vi "Main.vi"() -> ()   [LabVIEW 2013]
uses:
  ctl/config_ctl.ctl
  ctl/force_sensor_data.ctl
  ctl/UI_cmd-ctl.ctl
  ctl/file_path-cmd.ctl
  ctl/Data_analysis_mune_index.ctl
  <vilib>/Analysis/baseanly.llb/Mean (DBL).vi
  Global.vi
  <vilib>/Utility/file.llb/Read From Spreadsheet File (string).vi
  <vilib>/Analysis/NI_AALBase.lvlib
panel:
  out "simulation":bool=TRUE
  in  "sub_tab":enum32{"graph", "ref", "err"}(tab)=enum."ref"
  in  "Grapb_tap":enum32{"data graph", "sub graph"}(tab)=enum."sub graph"
  out "Strain chart w cal":waveform(dbl)[](graph)
  out "Force chart":waveform(dbl)(graph)
  out "vacuum chart":waveform(dbl)(graph)
  out "Heater chart":i32(graph)=2147483647
  out "Strain raw chart":waveform(dbl)[](graph)=[{"t0"=timestamp(3479370102.41062 s since 1904-01-01), "dt"=0.00062, "Y"=[0.0, 0.0, 0.0, 0.0, 0.0, 0.0, 0.0, 0.0, 0.0, 0.0, 0.0, 0.0, 0.0, 0.0, 0.0, 0.0, 0.0, 0.0, 0.0, 0.0, 0.0, 0.0, 0.0, 0.0, 0.0, 0.0, 0.0, 0.0, 0.0, 0.0, 0.0, 0.0, 0.0, 0.0, 0.0, 0.0, 0.0, 0.0, 0.0, 0.0, 0.0, 0.0, 0.0, 0.0, 0.0, 0.0, 0.0, 0.0, 0.0, 0.0, 0.0, 0.0, 0.0, 0.0, 0.0, 0.0, 0.0, 0.0, 0.0, 0.0, 0.0, 0.0, 0.0, 0.0, 0.0, 0.0, 0.0, 0.0, 0.0, 0.0, 0.0, 0.0, 0.0, 0.0, 0.0, 0.0, 0.0, 0.0, 0.0, 0.0, 0.0, 0.0, 0.0, 0.0, 0.0, 0.0, 0.0, 0.0, 0.0, 0.0, 0.0, 0.0, 0.0, 0.0, 0.0, 0.0, 0.0, 0.0, 0.0, 0.0], "attributes"=variant("NI_ChannelName"=variant(string "변형률_0"), "NI_UnitDescription"=variant(string "Strain"))}, {"t0"=timestamp(3479370102.41062 s since 1904-01-01), "dt"=0.00062, "Y"=[0.0, 0.0, 0.0, 0.0, 0.0, 0.0, 0.0, 0.0, 0.0, 0.0, 0.0, 0.0, 0.0, 0.0, 0.0, 0.0, 0.0, 0.0, 0.0, 0.0, 0.0, 0.0, 0.0, 0.0, 0.0, 0.0, 0.0, 0.0, 0.0, 0.0, 0.0, 0.0, 0.0, 0.0, 0.0, 0.0, 0.0, 0.0, 0.0, 0.0, 0.0, 0.0, 0.0, 0.0, 0.0, 0.0, 0.0, 0.0, 0.0, 0.0, 0.0, 0.0, 0.0, 0.0, 0.0, 0.0, 0.0, 0.0, 0.0, 0.0, 0.0, 0.0, 0.0, 0.0, 0.0, 0.0, 0.0, 0.0, 0.0, 0.0, 0.0, 0.0, 0.0, 0.0, 0.0, 0.0, 0.0, 0.0, 0.0, 0.0, 0.0, 0.0, 0.0, 0.0, 0.0, 0.0, 0.0, 0.0, 0.0, 0.0, 0.0, 0.0, 0.0, 0.0, 0.0, 0.0, 0.0, 0.0, 0.0, 0.0], "attributes"=variant("NI_ChannelName"=variant(string "변형률_1"), "NI_UnitDescription"=variant(string "Strain"))}, {"t0"=timestamp(3479370102.41062 s since 1904-01-01), "dt"=0.00062, "Y"=[0.0, 0.0, 0.0, 0.0, 0.0, 0.0, 0.0, 0.0, 0.0, 0.0, 0.0, 0.0, 0.0, 0.0, 0.0, 0.0, 0.0, 0.0, 0.0, 0.0, 0.0, 0.0, 0.0, 0.0, 0.0, 0.0, 0.0, 0.0, 0.0, 0.0, 0.0, 0.0, 0.0, 0.0, 0.0, 0.0, 0.0, 0.0, 0.0, 0.0, 0.0, 0.0, 0.0, 0.0, 0.0, 0.0, 0.0, 0.0, 0.0, 0.0, 0.0, 0.0, 0.0, 0.0, 0.0, 0.0, 0.0, 0.0, 0.0, 0.0, 0.0, 0.0, 0.0, 0.0, 0.0, 0.0, 0.0, 0.0, 0.0, 0.0, 0.0, 0.0, 0.0, 0.0, 0.0, 0.0, 0.0, 0.0, 0.0, 0.0, 0.0, 0.0, 0.0, 0.0, 0.0, 0.0, 0.0, 0.0, 0.0, 0.0, 0.0, 0.0, 0.0, 0.0, 0.0, 0.0, 0.0, 0.0, 0.0, 0.0], "attributes"=variant("NI_ChannelName"=variant(string "변형률_2"), "NI_UnitDescription"=variant(string "Strain"))}, {"t0"=timestamp(3479370102.41062 s since 1904-01-01), "dt"=0.00062, "Y"=[0.0, 0.0, 0.0, 0.0, 0.0, 0.0, 0.0, 0.0, 0.0, 0.0, 0.0, 0.0, 0.0, 0.0, 0.0, 0.0, 0.0, 0.0, 0.0, 0.0, 0.0, 0.0, 0.0, 0.0, 0.0, 0.0, 0.0, 0.0, 0.0, 0.0, 0.0, 0.0, 0.0, 0.0, 0.0, 0.0, 0.0, 0.0, 0.0, 0.0, 0.0, 0.0, 0.0, 0.0, 0.0, 0.0, 0.0, 0.0, 0.0, 0.0, 0.0, 0.0, 0.0, 0.0, 0.0, 0.0, 0.0, 0.0, 0.0, 0.0, 0.0, 0.0, 0.0, 0.0, 0.0, 0.0, 0.0, 0.0, 0.0, 0.0, 0.0, 0.0, 0.0, 0.0, 0.0, 0.0, 0.0, 0.0, 0.0, 0.0, 0.0, 0.0, 0.0, 0.0, 0.0, 0.0, 0.0, 0.0, 0.0, 0.0, 0.0, 0.0, 0.0, 0.0, 0.0, 0.0, 0.0, 0.0, 0.0, 0.0], "attributes"=variant("NI_ChannelName"=variant(string "변형률_3"), "NI_UnitDescription"=variant(string "Strain"))}]
  out "Strain raw graph":waveform(dbl)[](graph)=[{"t0"=timestamp(3479370102.41062 s since 1904-01-01), "dt"=0.00062, "Y"=[0.04635468247337127, 0.04635468247337127, 0.04635468247337127, 0.04635468247337127, 0.04635468247337127, 0.04635468247337127, 0.04635468247337127, 0.04635468247337127, 0.04635468247337127, 0.04635468247337127, 0.04635468247337127, 0.04635468247337127, 0.04635468247337127, 0.04635468247337127, 0.04635468247337127, 0.04635468247337127, 0.04635468247337127, 0.04635468247337127, 0.04635468247337127, 0.04635468247337127, 0.04635468247337127, 0.04635468247337127, 0.04635468247337127, 0.04635468247337127, 0.04635468247337127, 0.04635468247337127, 0.04635468247337127, 0.04635468247337127, 0.04635468247337127, 0.04635468247337127, 0.04635468247337127, 0.04635468247337127, 0.04635468247337127, 0.04635468247337127, 0.04635468247337127, 0.04635468247337127, 0.04635468247337127, 0.04635468247337127, 0.04635468247337127, 0.04635468247337127, 0.04635468247337127, 0.04635468247337127, 0.04635468247337127, 0.04635468247337127, 0.04635468247337127, 0.04635468247337127, 0.04635468247337127, 0.04635468247337127, 0.04635468247337127, 0.04635468247337127, 0.04635468247337127, 0.04635468247337127, 0.04635468247337127, 0.04635468247337127, 0.04635468247337127, 0.04635468247337127, 0.04635468247337127, 0.04635468247337127, 0.04635468247337127, 0.04635468247337127, 0.04635468247337127, 0.04635468247337127, 0.04635468247337127, 0.04635468247337127, 0.04635468247337127, 0.04635468247337127, 0.04635468247337127, 0.04635468247337127, 0.04635468247337127, 0.04635468247337127, 0.04635468247337127, 0.04635468247337127, 0.04635468247337127, 0.04635468247337127, 0.04635468247337127, 0.04635468247337127, 0.04635468247337127, 0.04635468247337127, 0.04635468247337127, 0.04635468247337127, 0.04635468247337127, 0.04635468247337127, 0.04635468247337127, 0.04635468247337127, 0.04635468247337127, 0.04635468247337127, 0.04635468247337127, 0.04635468247337127, 0.04635468247337127, 0.04635468247337127, 0.04635468247337127, 0.04635468247337127, 0.04635468247337127, 0.04635468247337127, 0.04635468247337127, 0.04635468247337127, 0.04635468247337127, 0.04635468247337127, 0.04635468247337127, 0.04635468247337127], "attributes"=variant("NI_ChannelName"=variant(string "변형률_0"), "NI_UnitDescription"=variant(string "Strain"))}, {"t0"=timestamp(3479370102.41062 s since 1904-01-01), "dt"=0.00062, "Y"=[0.04702815089622699, 0.04702815089622699, 0.04702815089622699, 0.04702815089622699, 0.04702815089622699, 0.04702815089622699, 0.04702815089622699, 0.04702815089622699, 0.04702815089622699, 0.04702815089622699, 0.04702815089622699, 0.04702815089622699, 0.04702815089622699, 0.04702815089622699, 0.04702815089622699, 0.04702815089622699, 0.04702815089622699, 0.04702815089622699, 0.04702815089622699, 0.04702815089622699, 0.04702815089622699, 0.04702815089622699, 0.04702815089622699, 0.04702815089622699, 0.04702815089622699, 0.04702815089622699, 0.04702815089622699, 0.04702815089622699, 0.04702815089622699, 0.04702815089622699, 0.04702815089622699, 0.04702815089622699, 0.04702815089622699, 0.04702815089622699, 0.04702815089622699, 0.04702815089622699, 0.04702815089622699, 0.04702815089622699, 0.04702815089622699, 0.04702815089622699, 0.04702815089622699, 0.04702815089622699, 0.04702815089622699, 0.04702815089622699, 0.04702815089622699, 0.04702815089622699, 0.04702815089622699, 0.04702815089622699, 0.04702815089622699, 0.04702815089622699, 0.04702815089622699, 0.04702815089622699, 0.04702815089622699, 0.04702815089622699, 0.04702815089622699, 0.04702815089622699, 0.04702815089622699, 0.04702815089622699, 0.04702815089622699, 0.04702815089622699, 0.04702815089622699, 0.04702815089622699, 0.04702815089622699, 0.04702815089622699, 0.04702815089622699, 0.04702815089622699, 0.04702815089622699, 0.04702815089622699, 0.04702815089622699, 0.04702815089622699, 0.04702815089622699, 0.04702815089622699, 0.04702815089622699, 0.04702815089622699, 0.04702815089622699, 0.04702815089622699, 0.04702815089622699, 0.04702815089622699, 0.04702815089622699, 0.04702815089622699, 0.04702815089622699, 0.04702815089622699, 0.04702815089622699, 0.04702815089622699, 0.04702815089622699, 0.04702815089622699, 0.04702815089622699, 0.04702815089622699, 0.04702815089622699, 0.04702815089622699, 0.04702815089622699, 0.04702815089622699, 0.04702815089622699, 0.04702815089622699, 0.04702815089622699, 0.04702815089622699, 0.04702815089622699, 0.04702815089622699, 0.04702815089622699, 0.04702815089622699], "attributes"=variant("NI_ChannelName"=variant(string "변형률_1"), "NI_UnitDescription"=variant(string "Strain"))}, {"t0"=timestamp(3479370102.41062 s since 1904-01-01), "dt"=0.00062, "Y"=[0.046751224408544026, 0.046751224408544026, 0.046751224408544026, 0.046751224408544026, 0.046751224408544026, 0.046751224408544026, 0.046751224408544026, 0.046751224408544026, 0.046751224408544026, 0.046751224408544026, 0.046751224408544026, 0.046751224408544026, 0.046751224408544026, 0.046751224408544026, 0.046751224408544026, 0.046751224408544026, 0.046751224408544026, 0.046751224408544026, 0.046751224408544026, 0.046751224408544026, 0.046751224408544026, 0.046751224408544026, 0.046751224408544026, 0.046751224408544026, 0.046751224408544026, 0.046751224408544026, 0.046751224408544026, 0.046751224408544026, 0.046751224408544026, 0.046751224408544026, 0.046751224408544026, 0.046751224408544026, 0.046751224408544026, 0.046751224408544026, 0.046751224408544026, 0.046751224408544026, 0.046751224408544026, 0.046751224408544026, 0.046751224408544026, 0.046751224408544026, 0.046751224408544026, 0.046751224408544026, 0.046751224408544026, 0.046751224408544026, 0.046751224408544026, 0.046751224408544026, 0.046751224408544026, 0.046751224408544026, 0.046751224408544026, 0.046751224408544026, 0.046751224408544026, 0.046751224408544026, 0.046751224408544026, 0.046751224408544026, 0.046751224408544026, 0.046751224408544026, 0.046751224408544026, 0.046751224408544026, 0.046751224408544026, 0.046751224408544026, 0.046751224408544026, 0.046751224408544026, 0.046751224408544026, 0.046751224408544026, 0.046751224408544026, 0.046751224408544026, 0.046751224408544026, 0.046751224408544026, 0.046751224408544026, 0.046751224408544026, 0.046751224408544026, 0.046751224408544026, 0.046751224408544026, 0.046751224408544026, 0.046751224408544026, 0.046751224408544026, 0.046751224408544026, 0.046751224408544026, 0.046751224408544026, 0.046751224408544026, 0.046751224408544026, 0.046751224408544026, 0.046751224408544026, 0.046751224408544026, 0.046751224408544026, 0.046751224408544026, 0.046751224408544026, 0.046751224408544026, 0.046751224408544026, 0.046751224408544026, 0.046751224408544026, 0.046751224408544026, 0.046751224408544026, 0.046751224408544026, 0.046751224408544026, 0.046751224408544026, 0.046751224408544026, 0.046751224408544026, 0.046751224408544026, 0.046751224408544026], "attributes"=variant("NI_ChannelName"=variant(string "변형률_2"), "NI_UnitDescription"=variant(string "Strain"))}, {"t0"=timestamp(3479370102.41062 s since 1904-01-01), "dt"=0.00062, "Y"=[0.04725649492680068, 0.04725649492680068, 0.04725649492680068, 0.04725649492680068, 0.04725649492680068, 0.04725649492680068, 0.04725649492680068, 0.04725649492680068, 0.04725649492680068, 0.04725649492680068, 0.04725649492680068, 0.04725649492680068, 0.04725649492680068, 0.04725649492680068, 0.04725649492680068, 0.04725649492680068, 0.04725649492680068, 0.04725649492680068, 0.04725649492680068, 0.04725649492680068, 0.04725649492680068, 0.04725649492680068, 0.04725649492680068, 0.04725649492680068, 0.04725649492680068, 0.04725649492680068, 0.04725649492680068, 0.04725649492680068, 0.04725649492680068, 0.04725649492680068, 0.04725649492680068, 0.04725649492680068, 0.04725649492680068, 0.04725649492680068, 0.04725649492680068, 0.04725649492680068, 0.04725649492680068, 0.04725649492680068, 0.04725649492680068, 0.04725649492680068, 0.04725649492680068, 0.04725649492680068, 0.04725649492680068, 0.04725649492680068, 0.04725649492680068, 0.04725649492680068, 0.04725649492680068, 0.04725649492680068, 0.04725649492680068, 0.04725649492680068, 0.04725649492680068, 0.04725649492680068, 0.04725649492680068, 0.04725649492680068, 0.04725649492680068, 0.04725649492680068, 0.04725649492680068, 0.04725649492680068, 0.04725649492680068, 0.04725649492680068, 0.04725649492680068, 0.04725649492680068, 0.04725649492680068, 0.04725649492680068, 0.04725649492680068, 0.04725649492680068, 0.04725649492680068, 0.04725649492680068, 0.04725649492680068, 0.04725649492680068, 0.04725649492680068, 0.04725649492680068, 0.04725649492680068, 0.04725649492680068, 0.04725649492680068, 0.04725649492680068, 0.04725649492680068, 0.04725649492680068, 0.04725649492680068, 0.04725649492680068, 0.04725649492680068, 0.04725649492680068, 0.04725649492680068, 0.04725649492680068, 0.04725649492680068, 0.04725649492680068, 0.04725649492680068, 0.04725649492680068, 0.04725649492680068, 0.04725649492680068, 0.04725649492680068, 0.04725649492680068, 0.04725649492680068, 0.04725649492680068, 0.04725649492680068, 0.04725649492680068, 0.04725649492680068, 0.04725649492680068, 0.04725649492680068, 0.04725649492680068], "attributes"=variant("NI_ChannelName"=variant(string "변형률_3"), "NI_UnitDescription"=variant(string "Strain"))}]
  out "Filtered force graph":waveform(dbl)[](graph)
  out "Force graph T":waveform(dbl)(graph)={"t0"=timestamp(0 s since 1904-01-01), "dt"=0.00062, "Y"=array[3100 elements]}
  out "error out UI":errorcluster caption="error out"
  in  "Data load":bool
  in  "Nulling":bool
  in  "pause":bool
  in  "START":bool
  in  "Main_tap":enum32{"Main", "Graph", "Load data", "Config"}(tab)
  out "Forece zoom Graph":dbl[](graph)
  out "simulation status":u32(slide) scale=0.0..4132.530364985612
  in  "Simulation config":cluster{"Raw data file path":path, "speed":u32}={"Raw data file path"=path "C:/FDCdata/data/*.dat", "speed"=10} {"speed" scale=0.0..100.0}
  out "Force graph T":waveform(dbl)(graph)={"t0"=timestamp(0 s since 1904-01-01), "dt"=0.00062, "Y"=array[4800 elements]}
  out "trigger":bool
  out "Pickup force":dbl=98.25510170952174 caption="Pickup force (g)" format="%.1f"
  out "Pickup time":dbl=272.17999999999967 caption="Pickup time (ms)" format="%.1f"
  in  "Status":string="\r\n18:26:27 - system ini start\r\n18:26:27 - system ini finish\r\n18:26:30 - Simulation start\r\n18:27:05 - Program stop"
  out "Balance xy rt":cluster{"X":dbl, "Y":dbl}[](graph)
  out "Bonding force":dbl=992.5036050877534 caption="Bonding force (g)" format="%.1f"
  out "Bonding time":dbl=1024.8600000000001 caption="Bonding time (ms)" format="%.1f"
  out "Heater_rt":dbl=nan caption="Heater" format="%.1f"
  out "Vacuum_rt":dbl=nan caption="Vacuum rt" format="%.1f"
  out "Force rt":dbl caption="Force" format="%.1f"
  out "vacuum T":dbl=36.062310289230055 format="%.1f"
  out "Heater temp T":dbl=85.0 caption="Heater temp (dg)" format="%.1f"
  out "Tensile force":dbl=35.0820285944681 caption="Tensile force (g)" format="%.1f"
  out "Balance xy T":cluster{"X":dbl, "Y":dbl}[](graph)=[{"X"=-5.263322791327499, "Y"=0.7308526066053755}]
  in  "Graph tap":enum32{"All", "IR", "Balance"}(tab)
  out "Mixed signal":cluster{"force":dbl, "vacuum":dbl, "temp":dbl}(graph)={"force"=0.0, "vacuum"=nan, "temp"=0.0}
  out "IR Image":T1(plugin-control)
  out "ROI intensity":dbl[][](graph)=[[nan, nan, nan, nan], [nan, nan, nan, nan]]
  in  "Data_tap":enum32{"Table", "Graph"}(tab)
  out "Data Table":string[][](table)=[["989.722772 ", " 1018.660000 ", " 129.870977 ", " 275.900000 ", " 39.437574 ", " 0.007857", "-0.075730 ", " 0.031476 ", " 0.000000 ", ""], ["1035.064263 ", " 1026.720000 ", " 141.740749 ", " 279.000000 ", " 21.594200 ", " 0.064365", "-0.070932 ", " -0.026859 ", " 0.000000 ", ""], ["953.326654 ", " 1018.040000 ", " 144.008701 ", " 276.520000 ", " 19.439881 ", " 0.048826", "-0.083029 ", " 0.031694 ", " 0.000000 ", ""], ["979.122812 ", " 1027.960000 ", " 140.533487 ", " 275.900000 ", " 17.521738 ", " 0.005569", "-0.069651 ", " 0.008560 ", " 0.000000 ", ""], ["1043.949852 ", " 1042.840000 ", " 134.488977 ", " 275.900000 ", " 13.192071 ", " 0.021168", "-0.072055 ", " 0.031519 ", " 0.000000 ", ""], ["1071.984719 ", " 1048.420000 ", " 138.327061 ", " 275.280000 ", " 25.559397 ", " 0.035083", "-0.035856 ", " -0.018712 ", " 0.000000 ", ""], ["1046.754193 ", " 1028.580000 ", " 142.008722 ", " 275.900000 ", " 18.790541 ", " 0.050977", "-0.061814 ", " 0.072167 ", " 0.000000 ", ""], ["978.664436 ", " 1027.960000 ", " 136.487201 ", " 276.520000 ", " 9.468253 ", " -0.003054", "-0.055865 ", " 0.026074 ", " 0.000000 ", ""], ["976.067518 ", " 1033.540000 ", " 146.571229 ", " 276.520000 ", " 22.608603 ", " 0.020801", "-0.074720 ", " -0.001809 ", " 0.000000 ", ""], ["1056.774276 ", " 1018.660000 ", " 147.195488 ", " 273.420000 ", " 10.587437 ", " 0.032608", "-0.051327 ", " 0.007079 ", " 0.000000 ", ""], ["990.239962 ", " 1018.660000 ", " 112.936811 ", " 270.320000 ", " 42.850519 ", " 0.033952", "-0.070209 ", " 0.070206 ", " 0.000000 ", ""], ["936.169153 ", " 1018.660000 ", " 140.782457 ", " 272.800000 ", " 12.421586 ", " -0.020109", "-0.070449 ", " 0.014964 ", " 0.000000 ", ""], ["941.421956 ", " 1014.320000 ", " 149.172818 ", " 274.660000 ", " 26.213624 ", " -0.007032", "-0.073163 ", " 0.004508 ", " 0.000000 ", ""], ["1034.387749 ", " 1023.000000 ", " 138.956480 ", " 270.940000 ", " 11.759580 ", " 0.086476", "-0.084766 ", " 0.052867 ", " 0.000000 ", ""], ["996.857727 ", " 1021.760000 ", " 157.070597 ", " 274.040000 ", " 25.263497 ", " 0.047311", "-0.063551 ", " 0.014572 ", " 0.000000 ", ""], ["989.722772 ", " 1018.660000 ", " 129.870977 ", " 275.900000 ", " 39.437574 ", " 0.007857", "-0.075730 ", " 0.031476 ", " 0.000000 ", ""], ["1035.064263 ", " 1026.720000 ", " 141.740749 ", " 279.000000 ", " 21.594200 ", " 0.064365", "-0.070932 ", " -0.026859 ", " 0.000000 ", ""], ["953.326654 ", " 1018.040000 ", " 144.008701 ", " 276.520000 ", " 19.439881 ", " 0.048826", "-0.083029 ", " 0.031694 ", " 0.000000 ", ""], ["979.122812 ", " 1027.960000 ", " 140.533487 ", " 275.900000 ", " 17.521738 ", " 0.005569", "-0.069651 ", " 0.008560 ", " 0.000000 ", ""], ["1043.949852 ", " 1042.840000 ", " 134.488977 ", " 275.900000 ", " 13.192071 ", " 0.021168", "-0.072055 ", " 0.031519 ", " 0.000000 ", ""], ["1071.984719 ", " 1048.420000 ", " 138.327061 ", " 275.280000 ", " 25.559397 ", " 0.035083", "-0.035856 ", " -0.018712 ", " 0.000000 ", ""], ["1046.754193 ", " 1028.580000 ", " 142.008722 ", " 275.900000 ", " 18.790541 ", " 0.050977", "-0.061814 ", " 0.072167 ", " 0.000000 ", ""], ["978.664436 ", " 1027.960000 ", " 136.487201 ", " 276.520000 ", " 9.468253 ", " -0.003054", "-0.055865 ", " 0.026074 ", " 0.000000 ", ""], ["976.067518 ", " 1033.540000 ", " 146.571229 ", " 276.520000 ", " 22.608603 ", " 0.020801", "-0.074720 ", " -0.001809 ", " 0.000000 ", ""], ["1056.774276 ", " 1018.660000 ", " 147.195488 ", " 273.420000 ", " 10.587437 ", " 0.032608", "-0.051327 ", " 0.007079 ", " 0.000000 ", ""], ["990.239962 ", " 1018.660000 ", " 112.936811 ", " 270.320000 ", " 42.850519 ", " 0.033952", "-0.070209 ", " 0.070206 ", " 0.000000 ", ""], ["936.169153 ", " 1018.660000 ", " 140.782457 ", " 272.800000 ", " 12.421586 ", " -0.020109", "-0.070449 ", " 0.014964 ", " 0.000000 ", ""], ["941.421956 ", " 1014.320000 ", " 149.172818 ", " 274.660000 ", " 26.213624 ", " -0.007032", "-0.073163 ", " 0.004508 ", " 0.000000 ", ""], ["1034.387749 ", " 1023.000000 ", " 138.956480 ", " 270.940000 ", " 11.759580 ", " 0.086476", "-0.084766 ", " 0.052867 ", " 0.000000 ", ""], ["996.857727 ", " 1021.760000 ", " 157.070597 ", " 274.040000 ", " 25.263497 ", " 0.047311", "-0.063551 ", " 0.014572 ", " 0.000000 ", ""]]
  out "Data result":cluster{"Mean":dbl, "Max":dbl, "Min":dbl}
  in  "Data menu":T2
  out "Load data":dbl[](graph)
  in  "file path":path=path "C:/FDCdata/data/Txt-data_1429_via_simulation.txt" caption="Data file path"
  in  "Load_setting":bool
  in  "Save_setting":bool
  in  "config tap":enum32{"Program", "Sensor"}(tab)
  in  "Config":T3={"Lower Cut-Off"=36.0, "Vacuum Trigger level"=20.0, "state settings"={"method"=enum."histogram", "histogram size"=512, "histogram method"=enum."mode", "reserved"=1.0}, "SPA-300 Setting"={"Bonding force (g)"=1000.0, "Bonding time (ms)"=1000.0, "Pickup force (g)"=100.0, "Pickup time (ms)"=500.0, "Speed"=enum."Slow"}} {"state settings"."reserved" format="%0.2f"}
  out "ROI":T4={"Global Rectangle"=[33, 12, 77, 40], "Contours"=[{"Contour Type"=0, "ROI Type"=3, "Points"=[33, 12, 77, 40]}]}
  in  "sensor data file path":path=path "C:/FDCdata/sensor/FS001002.dat"
  out "Force Sensor data":T5
  in  "Load sensor data":bool
  in  "정지":bool=TRUE
  # "DIE Attach Machine Monitoring"
  # "Real Monitoring"
  # "Balance"
  # "Force"
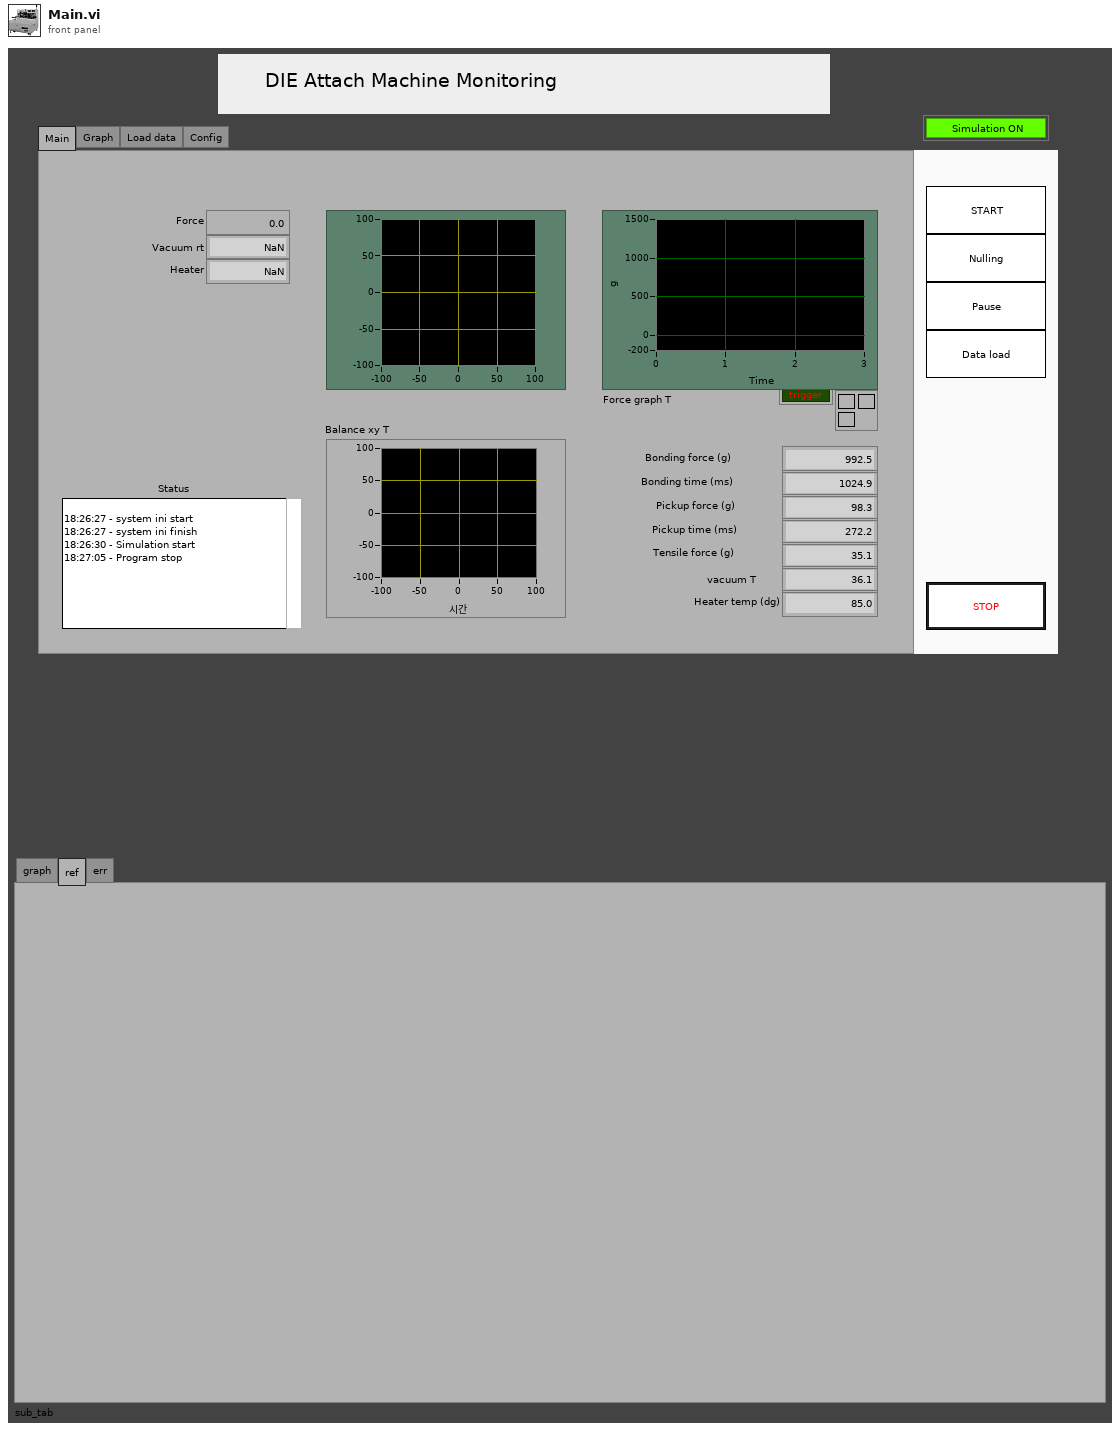
[diagram p1: front panel]
types:
  T1 = typedef "IMAQ Image.ctl" = refnum<image>
  T2 = cluster{"Force load":bool, "Force load 2":bool, "Force load 3":bool, "Force load 4":bool, "Force load 5":bool, "Force load 8":bool, "Force load 9":bool, "Force load 6":bool, "Force load 7":bool}
  T3 = typedef "config_ctl.ctl" = cluster{"Lower Cut-Off":dbl, "Vacuum Trigger level":dbl, "state settings":cluster{"method":enum32{"histogram", "peak", "auto select"}, "histogram size":i32, "histogram method":enum16{"mode"}, "reserved":dbl}, "SPA-300 Setting":cluster{"Bonding force (g)":dbl, "Bonding time (ms)":dbl, "Pickup force (g)":dbl, "Pickup time (ms)":dbl, "Speed":enum16{"Slow", "Fast"}}}
  T4 = cluster{"Global Rectangle":i32[], "Contours":cluster{"Contour Type":u32, "ROI Type":u32, "Points":i32[]}[]}
  T5 = typedef "force_sensor_data.ctl" = cluster{"weight":cluster{"front":dbl, "left":dbl, "back":dbl, "right":dbl}, "strain map":cluster{"x":dbl, "y":dbl}[]}
  T6 = typedef "UI_cmd-ctl.ctl" = enum16{"default", "create", "read"}
  T7 = enum8{"Enabled", "Disabled", "Disabled and Grayed Out"}
  T8 = cluster{"Heater temp T":refnum<vi>, "Heater chart":refnum<vi>, "vacuum T":refnum<vi>, "Balance xy rt":refnum<vi>, "Strain chart w cal":refnum<vi>, "Pickup force":refnum<vi>, "Pickup time":refnum<vi>, "Force chart":refnum<vi>, "Force graph T":refnum<vi>, "vacuum chart":refnum<vi>, "vacuum rt":refnum<vi>, "Strain raw graph":refnum<vi>, "Strain raw chart":refnum<vi>, "Bonding time":refnum<vi>, "Bonding force":refnum<vi>, "Balance xy T":refnum<vi>, "Filtered force graph":refnum<vi>, "ROI intensity":refnum<vi>, "Heater_rt":refnum<vi>, "Tensile force":refnum<vi>, "Force rt":refnum<vi>, "Mixed signal":refnum<vi>}
  T9 = typedef "q_data.ctl" = cluster{"Strain raw wf":waveform(dbl)[], "vacuum raw wf":waveform(dbl), "IR raw 2d":i16[][]}
  T10 = typedef "log_data.ctl" = cluster{"strain filter_n_nulling wf":waveform(dbl)[], "force wf":waveform(dbl), "force":dbl, "Balance xy wfs":cluster{"X":dbl, "Y":dbl}[], "vacuum kpa wf":waveform(dbl), "pcb temp":dbl[][]}
  T11 = typedef "file_path-cmd.ctl" = enum16{"default", "write"}
  T12 = typedef "Data_analysis_mune_index.ctl" = enum16{"Bonding Force", "Bonding Time", "Pickup Force", "Pickup Time", "Tensile Force", "Balance", "Vacuum", "Temperature"}
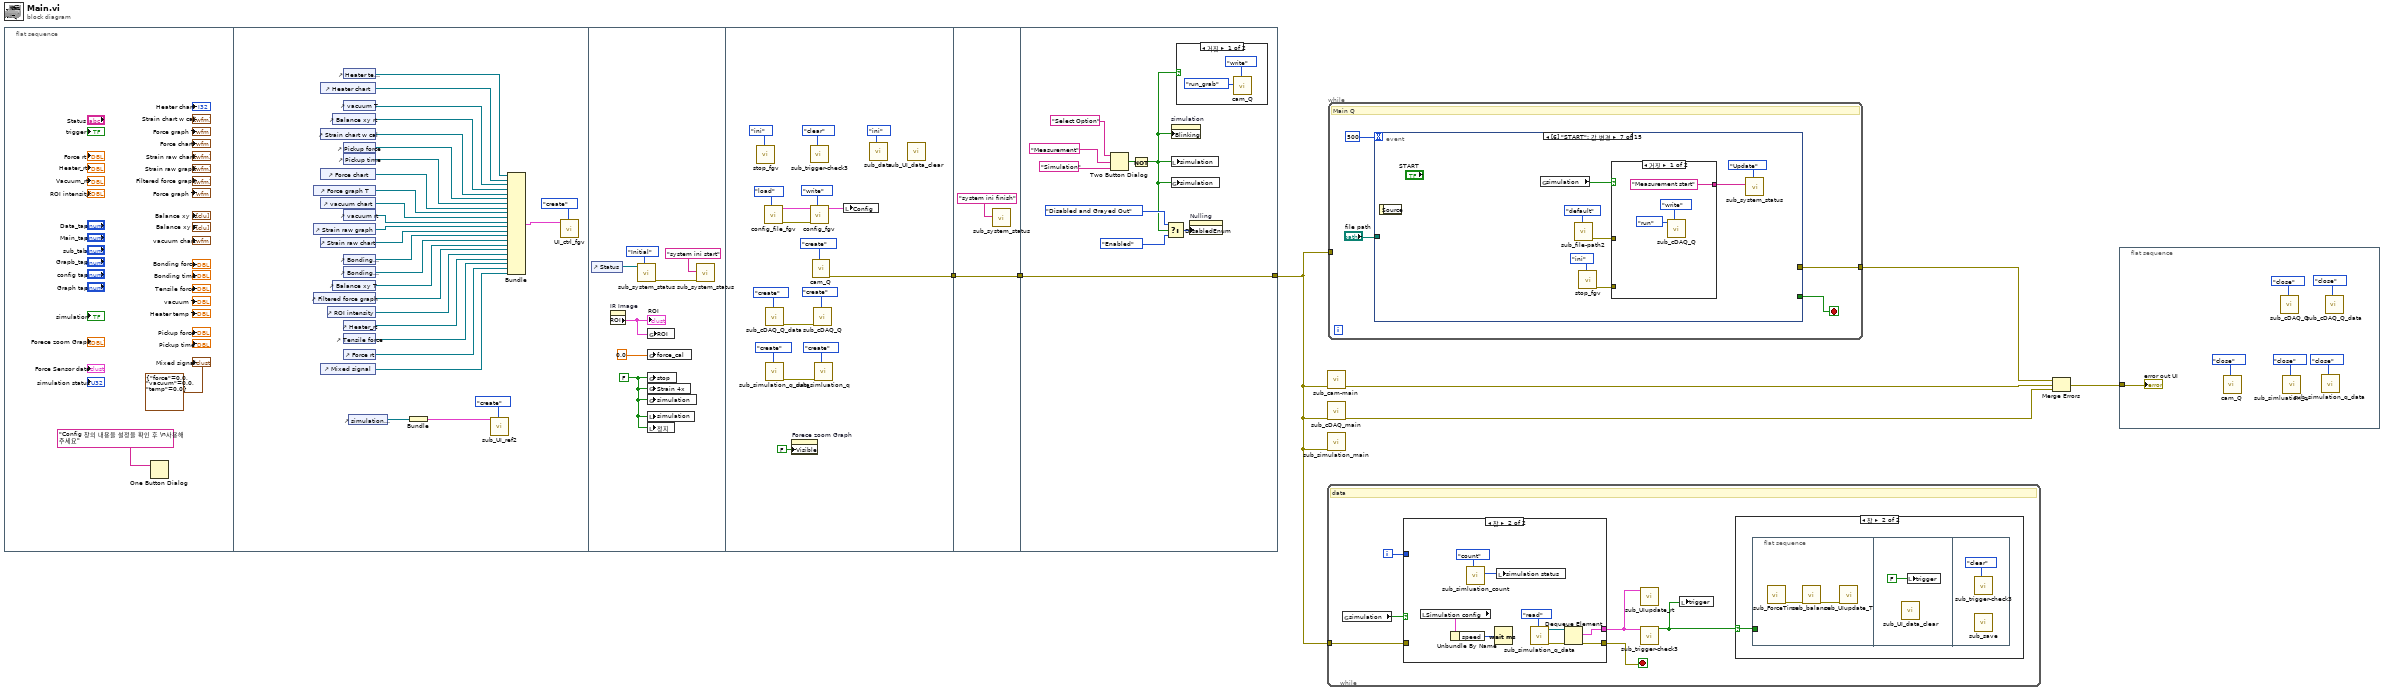
[diagram p0: block diagram]
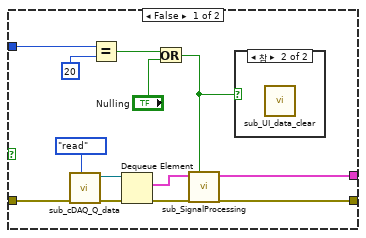
[diagram p2: hidden frame]
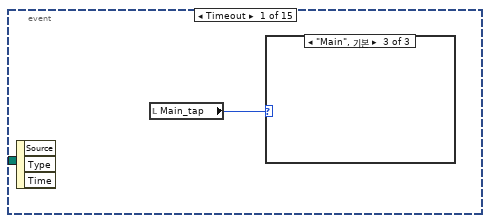
[diagram p5: hidden frame]
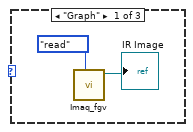
[diagram p6: hidden frame]
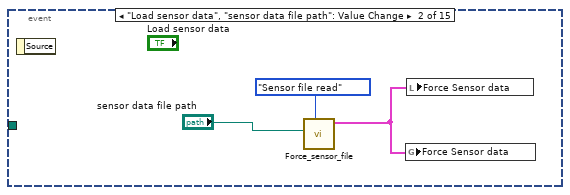
[diagram p8: hidden frame]
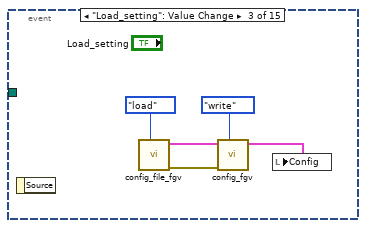
[diagram p9: hidden frame]
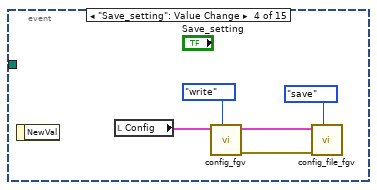
[diagram p10: hidden frame]
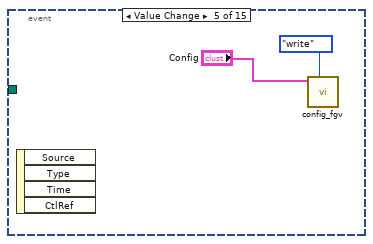
[diagram p11: hidden frame]
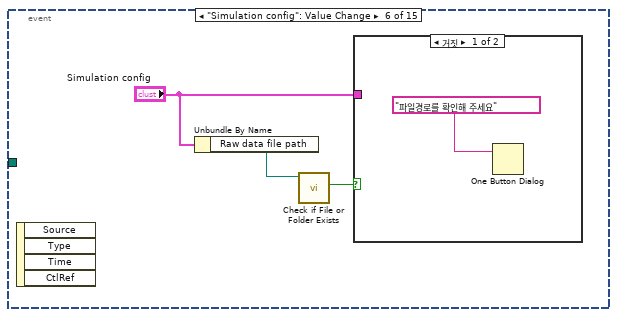
[diagram p12: hidden frame]
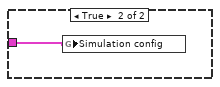
[diagram p13: hidden frame]
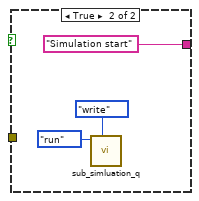
[diagram p14: hidden frame]
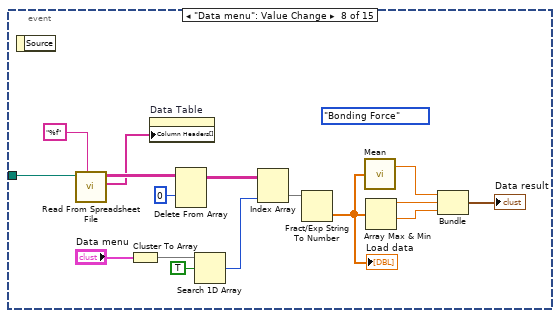
[diagram p15: hidden frame]
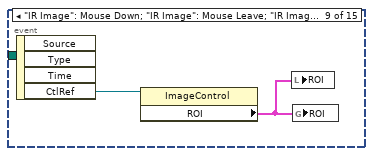
[diagram p16: hidden frame]
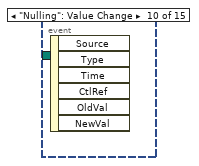
[diagram p17: hidden frame]
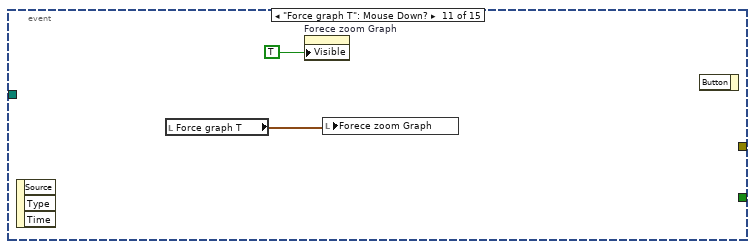
[diagram p18: hidden frame]
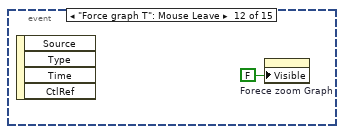
[diagram p19: hidden frame]
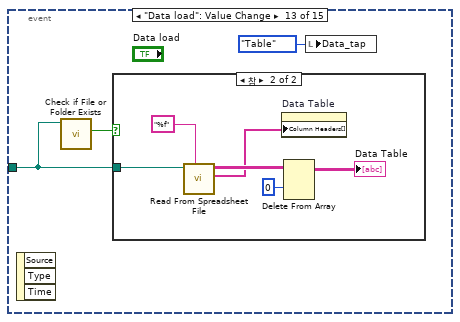
[diagram p20: hidden frame]
diagram:
  n1 = flat-sequence {
    tunnel: [w51] -> w7
    tunnel: w7 -> [w62]
    tunnel: [w62] -> w3
    tunnel: [w71] -> w4
    tunnel: w3 -> [w71]
    frame #0 {
      n2 = One Button Dialog(message="Config 창의 내용을 설정을 확인 후 \n사용해 주세요" ("버튼 이름(\"확인\")")) -> ()  [unwired: 1 in, 1 out]
      "Mixed signal" <- cluster{"force":dbl, "vacuum":dbl, "temp":dbl} {"force"=0.0, "vacuum"=0.0, "temp"=0.0}
    }
    frame #1 {
      n3 = control-ref of="Force graph T"() -> (w24:refnum<vi>)
      n4 = control-ref of="Strain raw graph"() -> (w34:refnum<vi>)
      n5 = control-ref of="Filtered force graph"() -> (w29:refnum<vi>)
      n6 = control-ref of="Heater chart"() -> (w17:refnum<vi>)
      n7 = control-ref of="Strain chart w cal"() -> (w20:refnum<vi>)
      n8 = control-ref of="Force chart"() -> (w23:refnum<vi>)
      n9 = control-ref of="vacuum chart"() -> (w36:refnum<vi>)
      n10 = control-ref of="Strain raw chart"() -> (w33:refnum<vi>)
      n11 = control-ref of="Mixed signal"() -> (w14:refnum<vi>)
      n12 = control-ref of="ROI intensity"() -> (w27:refnum<vi>)
      n13 = control-ref of="Balance xy rt"() -> (w19:refnum<vi>)
      n14 = control-ref of="Balance xy T"() -> (w30:refnum<vi>)
      n15 = control-ref of="Heater temp T"() -> (w16:refnum<vi>)
      n16 = control-ref of="vacuum T"() -> (w18:refnum<vi>)
      n17 = control-ref of="Pickup force"() -> (w22:refnum<vi>)
      n18 = control-ref of="Pickup time"() -> (w21:refnum<vi>)
      n19 = control-ref of="vacuum rt"() -> (w35:refnum<vi>)
      n20 = control-ref of="Bonding time"() -> (w32:refnum<vi>)
      n21 = control-ref of="Bonding force"() -> (w31:refnum<vi>)
      n22 = control-ref of="Heater_rt"() -> (w28:refnum<vi>)
      n23 = control-ref of="Tensile force"() -> (w25:refnum<vi>)
      n24 = control-ref of="Force rt"() -> (w15:refnum<vi>)
      n25 = control-ref of="simulation status"() -> (w11:refnum<vi>)
      n26 = Bundle("simulation status"=w11) -> (w10:cluster{"simulation status":refnum<vi>})  [unwired: 1 in]
      n27 = call "sub_UI_ref2.vi"("cmd"=UI_cmd-ctl."create", "UI ctl2 in"=w10) -> ()  [unwired: 9 in, 1 out]
      n28 = Bundle("Heater temp T"=w16, "Heater chart"=w17, "vacuum T"=w18, "Balance xy rt"=w19, "Strain chart w cal"=w20, "Pickup force"=w22, "Pickup time"=w21, "Force chart"=w23, "Force graph T"=w24, "vacuum chart"=w36, "vacuum rt"=w35, "Strain raw graph"=w34, "Strain raw chart"=w33, "Bonding time"=w32, "Bonding force"=w31, "Balance xy T"=w30, "Filtered force graph"=w29, "ROI intensity"=w27, "Heater_rt"=w28, "Tensile force"=w25, "Force rt"=w15, "Mixed signal"=w14) -> (w13:T8)  [unwired: 1 in]
      n29 = call "UI_ctrl_fgv.vi"("cmd"=UI_cmd-ctl."create", "UI cluster in"=w13) -> ()  [unwired: 9 in, 1 out]
    }
    frame #2 {
      w37 = FALSE ("stop")
      n30 = control-ref of="Status"() -> (w42:refnum<vi>)
      n31 = property on="IR Image" class="ImageControl"() -> ("ROI"=w43:T4)  [unwired: 2 in, 2 out]
      "ROI" <- w43
      n32 = call "sub_system_status.vi"("Mode"=enum16{"Initial", "Update", "Clear"}."Initial", "System Log"=w42) -> ("에러 출력"=w40:errorcluster)  [unwired: 9 in]
      n33 = global write "Global.vi" "force_cal"(0.0 ("force_cal")) -> ()
      n34 = global write "Global.vi" "stop"(w37) -> ()
      n35 = global write "Global.vi" "Strain 4x"(w37) -> ()
      n36 = global write "Global.vi" "simulation"(w37) -> ()
      n37 = local write "simulation"(w37) -> ()
      n38 = local write "정지"(w37) -> ()
      n39 = global write "Global.vi" "ROI"(w43) -> ()
      n40 = call "sub_system_status.vi"("에러 입력(에러 없음)"=w40, "String in"="system ini start") -> ()  [unwired: 9 in, 1 out]
    }
    frame #3 {
      n41 = call "stop_fgv.vi"("cmd"=enum16{"default", "ini", "stop"}."ini") -> ()  [unwired: 9 in, 2 out]
      n42 = call "config_file_fgv.vi"("cmd"=enum16{"save", "load"}."load") -> ("error out"=w55:errorcluster, "var"=w54:T3)  [unwired: 8 in, 1 out]
      n43 = call "sub_cDAQ_Q_data.vi"("cmd"=enum16{"create", "wirte", "read", "close"}."create") -> ("error out"=w49:errorcluster)  [unwired: 9 in, 1 out]
      n44 = call "sub_simulation_q_data.vi"("cmd"=enum16{"create", "wirte", "read", "close"}."create") -> ("error out"=w44:errorcluster)  [unwired: 9 in, 1 out]
      n45 = property on="Forece zoom Graph" class="WFGraph (엄격한)"("Visible"=FALSE ("보이기")) -> ()  [unwired: 2 in, 2 out]
      n46 = call "sub_trigger-check3.vi"("cmd"=enum16{"check", "clear"}."clear") -> ()  [unwired: 10 in, 1 out]
      n47 = call "config_fgv.vi"("cmd"=enum16{"write", "read", "ini"}."write", "error in"=w55, "Config in"=w54) -> ("Config out"=w53:T3)  [unwired: 7 in, 1 out]
      n48 = call "cam_Q.vi"("cmd"=enum16{"create", "write", "read", "close"}."create") -> ("error out"=w51:errorcluster)  [unwired: 9 in, 1 out]
      n49 = call "sub_cDAQ_Q.vi"("cmd"=enum16{"create", "write", "read", "close"}."create", "error in"=w49) -> ()  [unwired: 8 in, 2 out]
      n50 = call "sub_simluation_q.vi"("cmd"=enum16{"create", "write", "read", "close"}."create", "error in"=w44) -> ()  [unwired: 8 in, 2 out]
      n51 = local write "Config"(w53) -> ()
      n52 = call "sub_data.vi"("cmd"=enum16{"ini", "write", "read"}."ini") -> ()  [unwired: 9 in, 2 out]
      n53 = call "sub_UI_data_clear.vi"() -> ()  [unwired: 12 in]
    }
    frame #4 {
      n54 = call "sub_system_status.vi"("String in"="system ini finish") -> ()  [unwired: 10 in, 1 out]
    }
    frame #5 {
      n55 = Two Button Dialog(message="Select Option" ("메시지"), 1:"Simulation" ("참 버튼 이름(\"확인\")"), 2:"Measurement" ("거짓 버튼 이름(\"취소\")")) -> (T button?=w67:bool)
      n56 = Not(x=w67) -> (.not. x?=w63:bool)
      n57 = Select(t=T7."Disabled and Grayed Out" ("비활성화"), s=w63, f=T7."Enabled" ("비활성화")) -> (s? t:f=w66:T7)
      n58 = property on="simulation" class="Bool (엄격한)"("Blinking"=w63) -> ()  [unwired: 2 in, 2 out]
      n59 = local write "simulation"(w63) -> ()
      n60 = global write "Global.vi" "simulation"(w63) -> ()
      n61 = case shown="거짓" w63 {
        frame False {
          n62 = call "cam_Q.vi"("cmd"=enum16{"create", "write", "read", "close"}."write", "data"=enum16{"run_grab", "stop"}."run_grab") -> ()  [unwired: 8 in, 2 out]
        }
        frame True {
        }
      }
      n63 = property on="Nulling" class="Bool"("DisabledEnum"=w66) -> ()  [unwired: 2 in, 2 out]
    }
  }
  n64 = call "sub_cam-main.vi"("error in"=w4) -> ("error out"=w2:errorcluster)  [unwired: 10 in]
  n65 = call "sub_cDAQ_main.vi"("error in"=w4) -> ("error out"=w1:errorcluster)  [unwired: 10 in]
  n66 = call "sub_simulation_main.vi"("error in"=w4) -> ()  [unwired: 10 in, 1 out]
  n67 = while {
    tunnel: w4 -> [w78]
    i -> [w77]
    stop <- w79 stop-if-true
    # "data"
    n68 = global read "Global.vi" "simulation"() -> (w74:bool)
    n69 = case shown="참" w74 {
      tunnel: [w91 w100] -> w79
      tunnel: w78 -> [w88 _]
      tunnel: w77 -> [w84 _]
      tunnel: [w82 w96] -> w75
      frame False {
        n70 = call "sub_cDAQ_Q_data.vi"("cmd"=enum16{"create", "wirte", "read", "close"}."read", "error in"=w88) -> ("error out"=w87:errorcluster, "queue out"=w89:refnum<queue>)  [unwired: 8 in]
        n71 = Equal?(x=w84, y=20) -> (x = y?=w85:bool)
        n72 = Dequeue Element(queue=w89, error in (no error)=w87) -> (element=w83:T9, error out=w91:errorcluster)  [unwired: 1 in, 2 out]
        n73 = Or(x=w85, y="Nulling") -> (x .or. y?=w80:bool)
        n74 = call "sub_SignalProcessing.vi"("nulling"=w80, "Q_data"=w83) -> ("log data"=w82:T10)  [unwired: 8 in, 1 out]
        n75 = case shown="참" w80 {
          frame False {
          }
          frame True {
            n76 = call "sub_UI_data_clear.vi"() -> ()  [unwired: 12 in]
          }
        }
      }
      frame True {
        n77 = local read "Simulation config"() -> (w95:cluster{"Raw data file path":path, "speed":u32})
        n78 = Unbundle By Name(w95) -> ("speed"=w94:u32)
        n79 = call "sub_simluation_count.vi"("cmd"=enum16{"ini", "count"}."count") -> ("current"=w92:i32)  [unwired: 9 in, 1 out]
        n80 = Wait (ms)(milliseconds to wait=w94) -> ()  [unwired: 1 out]
        n81 = local write "simulation status"(w92) -> ()
        n82 = call "sub_simulation_q_data.vi"("cmd"=enum16{"create", "wirte", "read", "close"}."read") -> ("error out"=w98:errorcluster, "queue out"=w97:refnum<queue>)  [unwired: 9 in]
        n83 = Dequeue Element(queue=w97, error in (no error)=w98) -> (element=w96:T10, error out=w100:errorcluster)  [unwired: 1 in, 2 out]
      }
    }
    n84 = call "sub_UIupdate_rt.vi"("log data"=w75) -> ()  [unwired: 11 in]
    n85 = call "sub_trigger-check3.vi"("log data"=w75) -> ("trigger"=w76:bool)  [unwired: 10 in]
    n86 = local write "trigger"(w76) -> ()
    n87 = case shown="참" w76 {
      selector: w76 -> [_ w101]
      frame False {
      }
      frame True {
        n88 = flat-sequence {
          tunnel: w101 -> [_]
          frame #0 {
            n89 = call "sub_ForceTime.vi"() -> ("error out"=w103:errorcluster)  [unwired: 10 in, 1 out]
            n90 = call "sub_balance.vi"("error in"=w103) -> ("error out"=w102:errorcluster)  [unwired: 9 in, 1 out]
            n91 = call "sub_UIupdate_T.vi"("error in"=w102) -> ()  [unwired: 10 in, 1 out]
          }
          frame #1 {
            n92 = call "sub_UI_data_clear.vi"() -> ()  [unwired: 12 in]
            n93 = local write "trigger"(FALSE ("trigger")) -> ()
          }
          frame #2 {
            n94 = call "sub_trigger-check3.vi"("cmd"=enum16{"check", "clear"}."clear") -> ()  [unwired: 10 in, 1 out]
            n95 = call "sub_save.vi"() -> ()  [unwired: 12 in]
          }
        }
      }
    }
  }
  n96 = while {
    tunnel: w4 -> [_]
    tunnel: [w108] -> w6
    stop <- w109 stop-if-true
    # "Main Q"
    n97 = event shown="[6] \"START\": 값 변경" {
      selector: _ -> [_ _ _ _ _ _ _ _ _ _ _ _ _ _ _]
      dyn-events: _ -> [_ _ _ _ _ _ _ _ _ _ _ _ _ _ _]
      timeout: 500 -> [_ _ _ _ _ _ _ _ _ _ _ _ _ _ _]
      tunnel: [_ _ _ _ _ _ _ _ _ _ _ _ _ w185 _] -> w109
      tunnel: [_ _ _ _ _ _ _ _ _ _ _ _ _ _ w188] -> w108
      tunnel: "file path" -> [_ _ _ _ _ _ _ w154 _ _ _ _ w168 _ _]
      event Timeout {
        n98 = event-data() -> ()  [unwired: 1 in, 3 out]
        n99 = local read "Main_tap"() -> (w110:enum32{"Main", "Graph", "Load data", "Config"})
        n100 = case shown="\"Main\", 기본" w110 {
          frame "Graph" {
            n101 = call "Imaq_fgv.vi"("cmd"=enum16{"create", "close", "read"}."read") -> ("New Image"=→"IR Image":T1)  [unwired: 9 in, 1 out]
          }
          frame "Load data" {
          }
          frame "Main", Default {
          }
        }
      }
      event "Load sensor data", "sensor data file path": Value Change {
        n102 = event-data() -> ()  [unwired: 1 in, 1 out]
        n103 = call "Force_sensor_file.vi"("cmd"=enum16{"Sensor file create", "Sensor file read"}."Sensor file read", "file path"="sensor data file path") -> ("Force Sensor data out"=w114:T5)  [unwired: 8 in, 1 out]
        n104 = global write "Global.vi" "Force Sensor data"(w114) -> ()
        n105 = local write "Force Sensor data"(w114) -> ()
      }
      event "Load_setting": Value Change {
        n106 = event-data() -> ()  [unwired: 1 in, 1 out]
        n107 = call "config_file_fgv.vi"("cmd"=enum16{"save", "load"}."load") -> ("error out"=w119:errorcluster, "var"=w118:T3)  [unwired: 8 in, 1 out]
        n108 = call "config_fgv.vi"("cmd"=enum16{"write", "read", "ini"}."write", "error in"=w119, "Config in"=w118) -> ("Config out"=w116:T3)  [unwired: 7 in, 1 out]
        n109 = local write "Config"(w116) -> ()
      }
      event "Save_setting": Value Change {
        n110 = event-data() -> ()  [unwired: 1 in, 1 out]
        n111 = local read "Config"() -> (w122:T3)
        n112 = call "config_fgv.vi"("cmd"=enum16{"write", "read", "ini"}."write", "Config in"=w122) -> ("error out"=w123:errorcluster, "Config out"=w121:T3)  [unwired: 8 in]
        n113 = call "config_file_fgv.vi"("cmd"=enum16{"save", "load"}."save", "error in"=w123, "Config"=w121) -> ()  [unwired: 6 in, 3 out]
      }
      event Value Change {
        n114 = event-data() -> ()  [unwired: 1 in, 4 out]
        n115 = call "config_fgv.vi"("cmd"=enum16{"write", "read", "ini"}."write", "Config in"="Config") -> ()  [unwired: 8 in, 2 out]
      }
      event "Simulation config": Value Change {
        n116 = event-data() -> ()  [unwired: 1 in, 4 out]
        n117 = Unbundle By Name("Simulation config") -> ("Raw data file path"=w130:path)
        n118 = call <vilib>:"Check if File or Folder Exists.vi"("path"=w130) -> ("file or folder exists?"=w129:bool)  [unwired: 8 in, 2 out]
        n119 = case shown="거짓" w129 {
          tunnel: "Simulation config" -> [_ w132]
          frame False {
            n120 = One Button Dialog(message="파일경로를 확인해 주세요" ("메시지")) -> ()  [unwired: 1 in, 1 out]
          }
          frame True {
            n121 = global write "Global.vi" "Simulation config"(w132) -> ()
          }
        }
      }
      event "START": Value Change {
        n122 = event-data() -> ()  [unwired: 1 in, 1 out]
        n123 = global read "Global.vi" "simulation"() -> (w135:bool)
        n124 = call "sub_file-path2.vi"("cmd"=file_path-cmd."default") -> ("error out"=w133:errorcluster)  [unwired: 8 in, 2 out]
        n125 = call "stop_fgv.vi"("cmd"=enum16{"default", "ini", "stop"}."ini") -> ("error out"=w136:errorcluster)  [unwired: 9 in, 1 out]
        n126 = case shown="거짓" w135 {
          tunnel: w136 -> [_ _]
          tunnel: ["Measurement start" ("String in") "Simulation start" ("String in")] -> w134
          tunnel: w133 -> [_ _]
          frame False {
            n127 = call "sub_cDAQ_Q.vi"("cmd"=enum16{"create", "write", "read", "close"}."write", "data"=enum16{"run", "stop"}."run") -> ()  [unwired: 8 in, 2 out]
          }
          frame True {
            n128 = call "sub_simluation_q.vi"("cmd"=enum16{"create", "write", "read", "close"}."write", "data"=enum16{"run", "stop"}."run") -> ()  [unwired: 8 in, 2 out]
          }
        }
        n129 = call "sub_system_status.vi"("Mode"=enum16{"Initial", "Update", "Clear"}."Update", "String in"=w134) -> ()  [unwired: 9 in, 1 out]
      }
      event "Data menu": Value Change {
        (unwired) Data_analysis_mune_index."Bonding Force"
        n130 = event-data() -> ()  [unwired: 1 in, 1 out]
        n131 = call-poly <vilib>:"Read From Spreadsheet File.vi"("format (%s)"="%f", "file path (dialog if empty)"=w154) -> ("first row"=w158:string[], "all rows"=w160:string[][])  [unwired: 5 in, 3 out]
        n132 = Cluster To Array(cluster="Data menu") -> (array=w156:bool[])
        n133 = property on="Data Table" class="Tbl (엄격한)"("Column Headers[]"=w158) -> ()  [unwired: 2 in, 2 out]
        n134 = Delete From Array(array=w160, index (row)=0 ("인덱스 (행)")) -> (array with subset deleted=w153:string[][])  [unwired: 2 in, 1 out]
        n135 = Search 1D Array(1D array=w156, element=TRUE ("원소")) -> (index of element=w152:i32)  [unwired: 1 in]
        n136 = Index Array(array=w153, index (col)=w152) -> (element=w151:string[])  [unwired: 1 in]
        n137 = Fract/Exp String To Number(string=w151) -> (number=w150:dbl[])  [unwired: 3 in, 1 out]
        "Load data" <- w150
        n138 = call-poly <vilib>:"Mean.vi"("X"=w150) -> ("mean"=w149:dbl)  [unwired: 1 out]
        n139 = Array Max & Min(array=w150) -> (max value=w148:dbl, min value=w147:dbl)  [unwired: 2 out]
        n140 = Bundle("mean"=w149, w148, w147) -> (→"Data result":cluster{"mean":dbl, dbl, dbl})  [unwired: 1 in]
      }
      event "IR Image": Mouse Down; "IR Image": Mouse Leave; "IR Image": Mouse Move {
        n141 = event-data() -> ("CtlRef"=w163:refnum<vi>)  [unwired: 1 in, 3 out]
        n142 = property class="ImageControl"(reference=w163) -> ("ROI"=w162:T4)  [unwired: 1 in, 2 out]
        n143 = local write "ROI"(w162) -> ()
        n144 = global write "Global.vi" "ROI"(w162) -> ()
      }
      event "Nulling": Value Change {
        n145 = event-data() -> ()  [unwired: 1 in, 6 out]
      }
      event "Force graph T": Mouse Down? {
        n146 = event-data() -> ()  [unwired: 1 in, 3 out]
        n147 = local read "Force graph T"() -> (w164:waveform(dbl))
        n148 = property on="Forece zoom Graph" class="WFGraph (엄격한)"("Visible"=TRUE ("보이기")) -> ()  [unwired: 2 in, 2 out]
        n149 = local write "Forece zoom Graph"(w164) -> ()
        n150 = event-data() -> ()  [unwired: 2 in, 1 out]
      }
      event "Force graph T": Mouse Leave {
        n151 = event-data() -> ()  [unwired: 1 in, 4 out]
        n152 = property on="Forece zoom Graph" class="WFGraph (엄격한)"("Visible"=FALSE ("보이기")) -> ()  [unwired: 2 in, 2 out]
      }
      event "Data load": Value Change {
        n153 = event-data() -> ()  [unwired: 1 in, 3 out]
        n154 = call <vilib>:"Check if File or Folder Exists.vi"("path"=w168) -> ("file or folder exists?"=w167:bool)  [unwired: 8 in, 2 out]
        n155 = case shown="참" w167 {
          tunnel: w168 -> [_ w171]
          frame False {
            n156 = One Button Dialog(message="파일경로를 재 설정해 주세요" ("메시지")) -> ()  [unwired: 1 in, 1 out]
          }
          frame True {
            n157 = call-poly <vilib>:"Read From Spreadsheet File.vi"("format (%s)"="%f", "file path (dialog if empty)"=w171) -> ("first row"=w172:string[], "all rows"=w175:string[][])  [unwired: 5 in, 3 out]
            n158 = property on="Data Table" class="Tbl (엄격한)"("Column Headers[]"=w172) -> ()  [unwired: 2 in, 2 out]
            n159 = Delete From Array(array=w175, index (row)=0 ("인덱스 (행)")) -> (array with subset deleted=→"Data Table":string[][])  [unwired: 2 in, 1 out]
          }
        }
        n160 = local write "Data_tap"(enum32{"Table", "Graph"}."Table" ("Data_tap")) -> ()
      }
      event "정지": Value Change {
        w185 = TRUE ("stop")
        n161 = event-data() -> ()  [unwired: 1 in, 1 out]
        n162 = call "stop_fgv.vi"("cmd"=enum16{"default", "ini", "stop"}."stop") -> ("error out"=w179:errorcluster)  [unwired: 9 in, 1 out]
        n163 = call "sub_simluation_q.vi"("cmd"=enum16{"create", "write", "read", "close"}."write", "data"=enum16{"run", "stop"}."stop") -> ()  [unwired: 8 in, 2 out]
        n164 = call "sub_cDAQ_Q.vi"("cmd"=enum16{"create", "write", "read", "close"}."write", "data"=enum16{"run", "stop"}."stop") -> ()  [unwired: 8 in, 2 out]
        n165 = call "cam_Q.vi"("cmd"=enum16{"create", "write", "read", "close"}."write", "error in"=w179, "data"=enum16{"run_grab", "stop"}."stop") -> ()  [unwired: 7 in, 2 out]
        n166 = global write "Global.vi" "stop"(w185) -> ()
        n167 = call "sub_system_status.vi"("String in"="Program stop") -> ()  [unwired: 10 in, 1 out]
      }
      event "pause": Value Change {
        n168 = event-data() -> ()  [unwired: 1 in, 6 out]
        n169 = property on="Nulling" class="Bool"("DisabledEnum"=T7."Enabled" ("비활성화")) -> ()  [unwired: 2 in, 2 out]
        n170 = call "stop_fgv.vi"("cmd"=enum16{"default", "ini", "stop"}."stop") -> ("error out"=w188:errorcluster)  [unwired: 9 in, 1 out]
      }
    }
  }
  n171 = Merge Errors(w6, w2, w1) -> (w5:errorcluster)
  n172 = flat-sequence {
    tunnel: w5 -> [w194]
    frame #0 {
      n173 = call "cam_Q.vi"("cmd"=enum16{"create", "write", "read", "close"}."close") -> ()  [unwired: 9 in, 2 out]
      n174 = call "sub_cDAQ_Q.vi"("cmd"=enum16{"create", "write", "read", "close"}."close") -> ()  [unwired: 9 in, 2 out]
      n175 = call "sub_simluation_q.vi"("cmd"=enum16{"create", "write", "read", "close"}."close") -> ()  [unwired: 9 in, 2 out]
      n176 = call "sub_simulation_q_data.vi"("cmd"=enum16{"create", "wirte", "read", "close"}."close") -> ()  [unwired: 9 in, 2 out]
      n177 = call "sub_cDAQ_Q_data.vi"("cmd"=enum16{"create", "wirte", "read", "close"}."close") -> ()  [unwired: 9 in, 2 out]
      "error out UI" <- w194
    }
  }
